vi "cloud.vi"() -> ()   [LabVIEW 2021]
uses:
  <vilib>/httpClient/POSTBuffer.vi
  <vilib>/httpClient/LabVIEWHTTPClient.lvlib
panel:
  in  "buffer":string
  out "concatenated string":string
  out "error out 2":errorcluster
  out "error out":errorcluster
  out "x+1":dbl
  in  "s":bool
  out "headers":string
  out "body":string
  in  "stop":bool
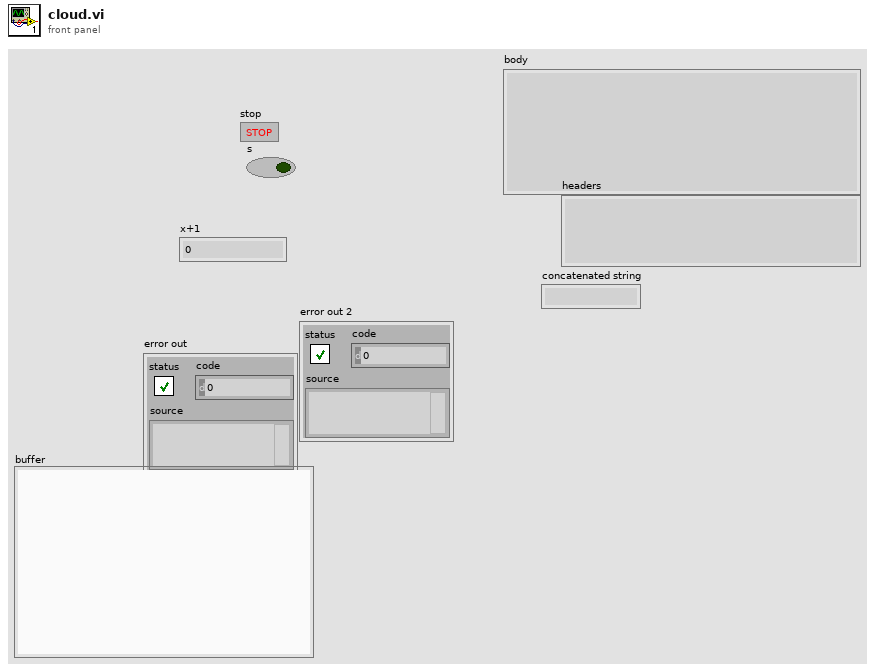
[diagram p1: front panel]
types:
  T1 = typedef "LabVIEWHTTPClient.lvlib/ClientHandle.ctl" = refnum<k1>
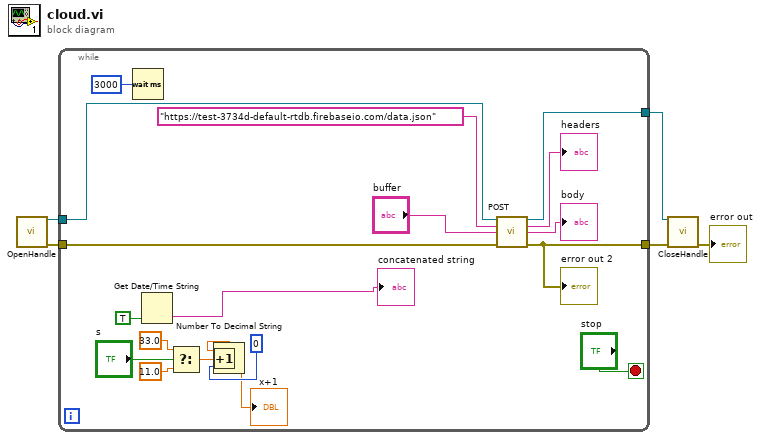
[diagram p0: block diagram]
diagram:
  n1 = call <vilib>:"OpenHandle.vi"() -> ("client handle out"=w5:T1, "error out"=w4:errorcluster)  [unwired: 14 in]
  n2 = while {
    tunnel: w5 -> [w22]
    tunnel: w4 -> [w21]
    tunnel: [w14] -> w3
    tunnel: [w13] -> w2
    stop <- "stop" stop-if-true
    n3 = Wait (ms)(milliseconds to wait=u32 3000) -> ()  [unwired: 1 out]
    n4 = Get Date/Time String(want seconds? (F)=TRUE) -> (time string=→"concatenated string":string)  [unwired: 2 in, 1 out]
    n5 = Select(t=33.0, s="s", f=11.0) -> (s? t:f=w18:dbl)
    n6 = Increment(x=w18) -> (x+1=w9:dbl)
    "x+1" <- w9
    n7 = Number To Decimal String(number=w9, width (-)=i16 0) -> ()  [unwired: 1 out]
    n8 = call-poly <vilib>:"POST.vi"("client handle"=w22, "url"="https://test-3734d-default-rtdb.firebaseio.com/data.json", "buffer"="buffer", "error in (no error)"=w21) -> ("client handle out"=w14:T1, "headers"=→"headers":string, "body"=→"body":string, "error out"=w13:errorcluster)  [unwired: 8 in]
    "error out 2" <- w13
  }
  n9 = call <vilib>:"CloseHandle.vi"("client handle"=w3, "error in (no error)"=w2) -> ("error out"=→"error out":errorcluster)  [unwired: 13 in]
